vi "TX_sequences.vi"(0 "error in (no error)":errorcluster, 2 "code":enum16{"无编码", "RS码", "卷积码"}(ring), 3 "输入要传输的信息":string="hello,my name is liuxiaowei. if you have any thing  please let me know!") -> (6 "signal for calculate ber":i8[](array[numeric]), 7 "error out":errorcluster, 8 "message_bit":i8[](array[numeric]), 9 "guard_bit":i8[](array[numeric]), 10 "syc bit":i8[](array[numeric]))   [LabVIEW 2010]
uses:
  <vilib>/addons/Modulation/Digital/General/MT Generate Bits (User Defined).vi
  <vilib>/addons/Modulation/niDMT.lvlib
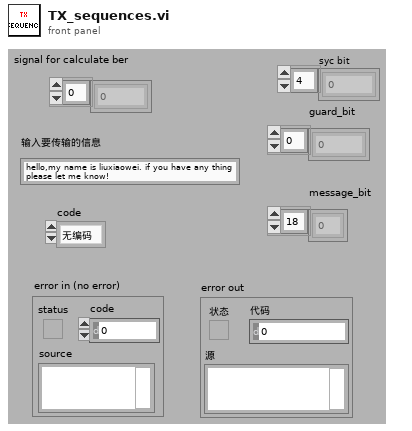
[diagram p1: front panel]
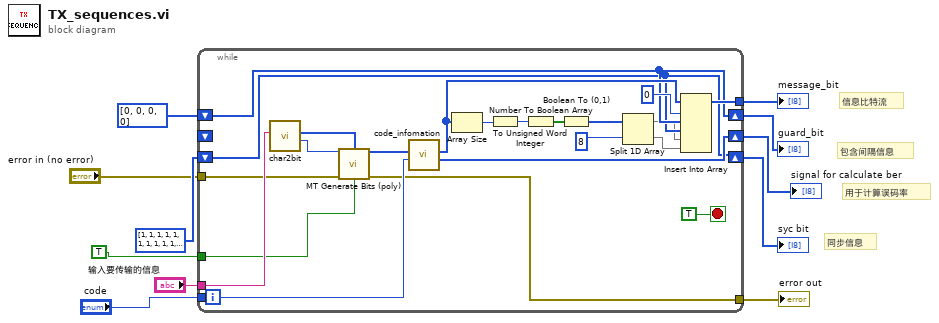
[diagram p0: block diagram]
diagram:
  # "信息比特流"
  # "包含间隔信息"
  # "用于计算误码率"
  # "同步信息"
  n1 = while {
    tunnel: "输入要传输的信息" -> [w33]
    tunnel: [w32] -> w10
    shift-right: [w17] -> w5
    shift-left: i8[] [1, 1, 1, 1, 1, 1, 1, 1, 1, 1, 1, 1, 1, 1, 1, 1] ("syn_bit") -> [w17]
    shift-right: [w18] -> w9
    shift-left: i8[] [0, 0, 0, 0] ("syn_bit") -> [w18]
    shift-right: [w30] -> w1
    shift-left: _ -> [_]
    tunnel: "code" -> [w29]
    tunnel: TRUE -> [w24]
    tunnel: [w19] -> w4
    tunnel: "error in (no error)" -> [w12]
    stop <- TRUE stop-if-true
    n2 = call "char2bit.vi"("输入要传输的信息"=w33) -> ("用户信息大小"=w27:i32, "输出比特信息"=w28:i8[])  [unwired: 9 in]
    n3 = call-poly <vilib>:"MT Generate Bits (poly).vi"("total bits (128)"=w27, "user base bit pattern"=w28, "error in (no error)"=w12, "reset? (T)"=w24) -> ("output bit stream"=w26:i8[], "error out"=w19:errorcluster)  [unwired: 10 in]
    n4 = call "code_infomation.vi"("code"=w29, "signal_in"=w26) -> ("signal_out_for_calclulate_ber"=w30:i8[], "signal_out_code"=w23:i8[])  [unwired: 8 in]
    n5 = Array Size(array=w23) -> (size(s)=w14:i32)
    n6 = To Unsigned Word Integer(number=w14) -> (unsigned 16bit integer=w13:u16)
    n7 = Number To Boolean Array(number=w13) -> (Boolean array=w22:bool[])
    n8 = Boolean To (0,1)(Boolean=w22) -> (0, 1=w21:i16[])
    n9 = Split 1D Array(array=w21, index=8 ("索引")) -> (first subarray=w16:i16[], second subarray=w15:i16[])
    n10 = Insert Into Array(array=w23, index=0 ("索引"), new element #1=w18, new element #2=w17, new element #3=w16, new element #4=w15) -> (w32:i8[])
  }
  "message_bit" <- w10
  "guard_bit" <- w9
  "error out" <- w4
  "signal for calculate ber" <- w1
  "syc bit" <- w5
